vi "xyzt-gui.vi"() -> ()   [LabVIEW 2011]
panel:
  in  "close":bool
  in  "Tab Control":enum32{"Setup", "Run"}(tab)
  in  "start":dbl=0.00262763 min=0.0 max=0.03 step=1e-06 format="%#_6p"
  in  "end":dbl=0.00275375 min=1e-06 max=0.03 step=1e-06 format="%#_6p"
  in  "distance":dbl=1e-05 min=0.0 max=0.0005 step=1e-07 format="%#_6p"
  out "Slices":u16=13
  in  "Get start":bool
  in  "Get end":bool
  in  "Power":T1={"Start-power"=0.02, "double distance"=0.0001} {"double distance" min=0.0 max=0.00025 step=1e-06 format="%#_6p"; "Start-power" format="%#_3p"}
  in  "Frame-time":dbl=1.61596
  in  "z-delay [s]":dbl=0.2 min=0.0 step=0.1
  in  "Get frametime":bool
  in  "xy-positions":dbl[][](array[numeric])=[[0.01555, 0.01516], [0.01923, 0.01332]]
  in  "move time [s]":dbl=2.0
  in  "Add current":bool
  in  "Motors":string[](array[string])=["stage.x", "stage.y"]
  in  "Time":dbl=60.0
  in  "Executions":u32=4
  in  "Calculate fastest":bool
  in  "Experiment-name":string="Z-xy-Time4"
  in  "Run":bool
  in  "cancel":bool
  out "Running":u16[](array[numeric])=[3, 1, 1]
  out "of":u32[](array[numeric])=[13, 2, 4]
  out "wait (time loop)":ext=52.08099985122681
  in  "runstate":enum16{"idle", "run", "cancel", "exit"}(ring)=enum."exit"
  # "First: z-stack"
  # "Second: position or filter"
  # "Third: time-loop"
  # "use u for µm, m for mm"
  # "empty = current only"
  # "Remove:\nRight click on row: Delete Row"
  # "z-loop\n\nmotor-loop\n\ntime-loop"
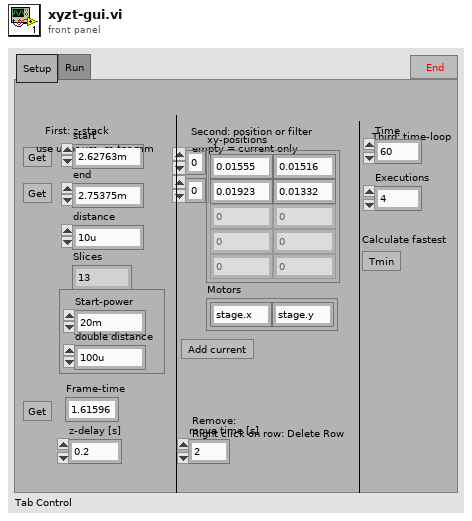
[diagram p1: front panel]
types:
  T1 = cluster{"Start-power":dbl, "double distance":dbl}
  T2 = enum16{"None/#Datasets", "Clear", "TagValueOf#", "AddValues", "ReadValue", "ChangeValue", "Get all"}
  T3 = typedef "ScanControl.ctl" = cluster{"Time [s]":dbl, "action":T4, "channel":T5, "value (/s)":dbl}[]
  T4 = typedef "ScanControl_Action.ctl" = enum16{"Abs", "Rel", "Inc", "IncInc", "LoopStart", "LoopEnd", "WaitTriggerRising"}
  T5 = typedef "ScanControl_Channel.ctl" = enum16{"Com", "AnalogConfig", "AnalogValue", "GalvoX", "GalvoY", "Galvo3", "Galvo4", "Digital", "Free", "Loop", "SMoveTime", "Image1X", "Image1Y", "Image2X", "Image2Y"}
  T6 = cluster{"Time [s]":dbl, "action":T4, "channel":T5, "value (/s)":dbl}
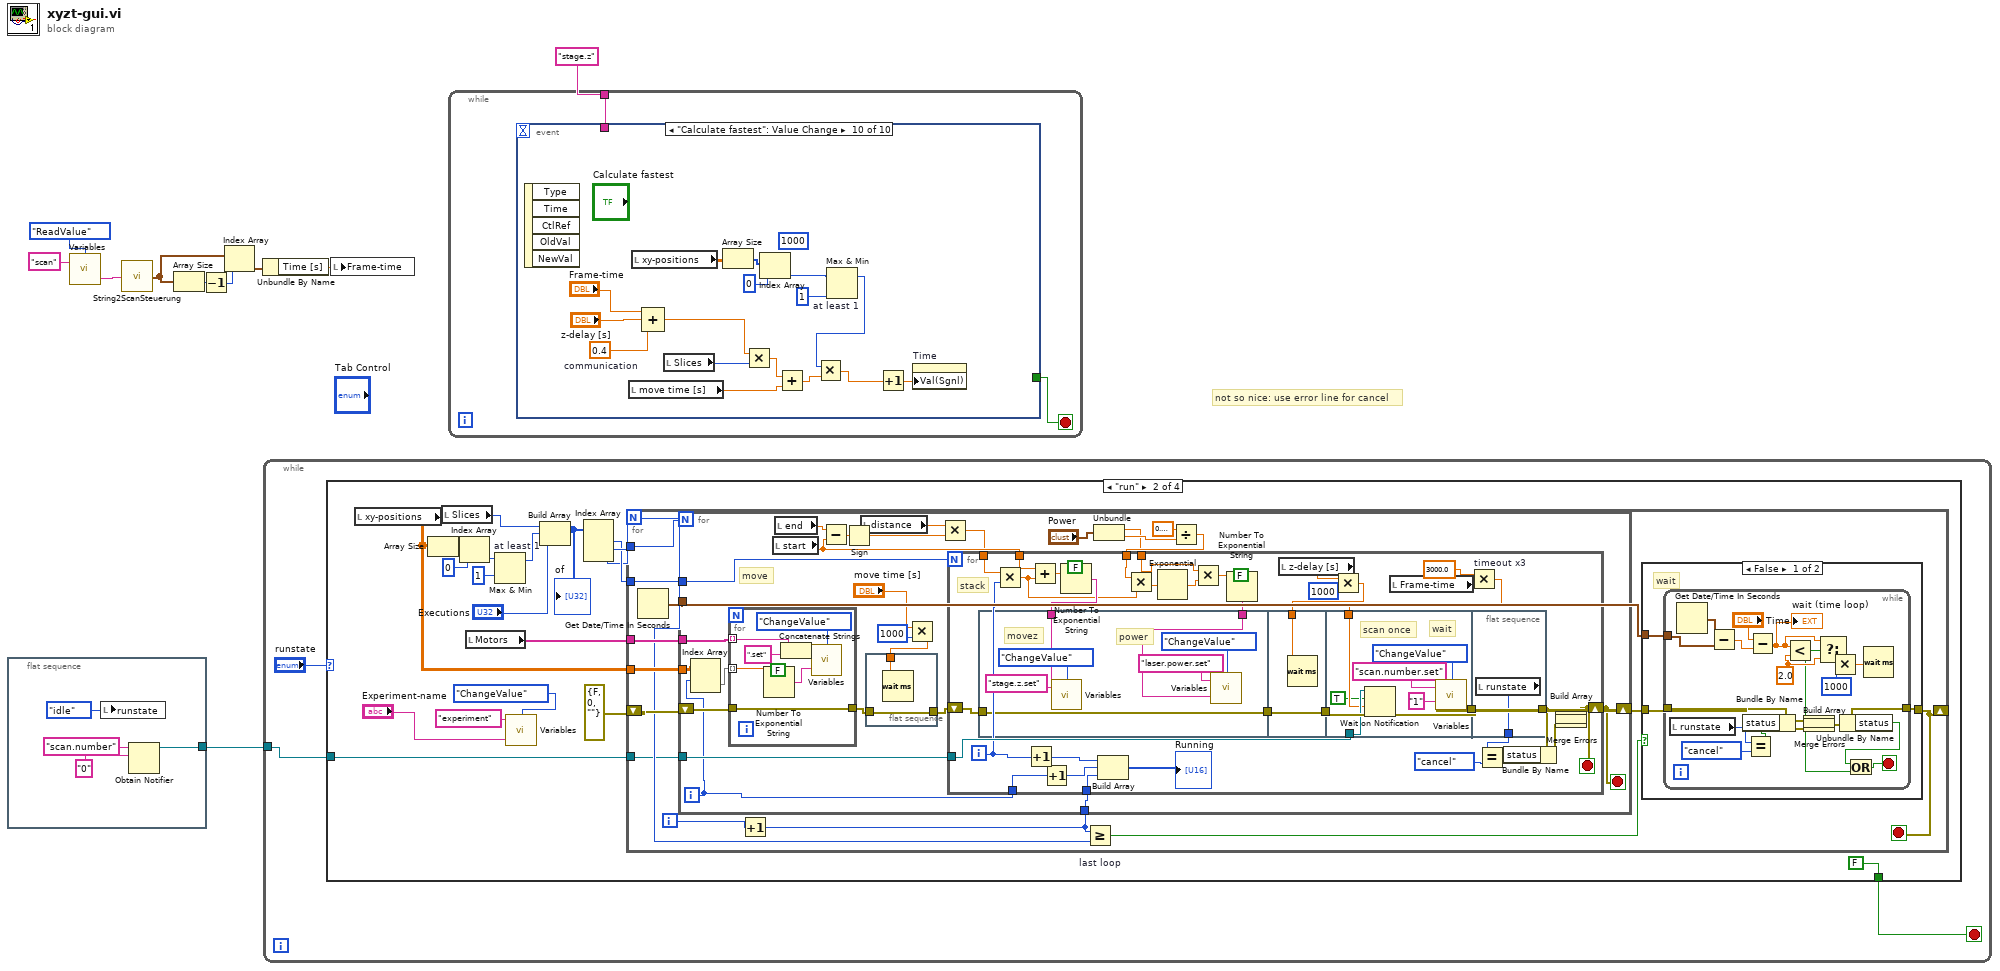
[diagram p0: block diagram]
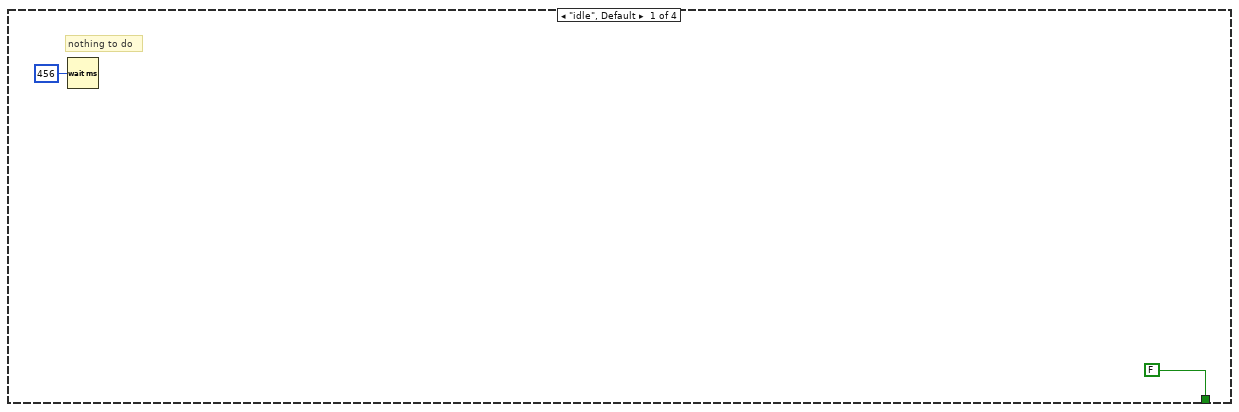
[diagram p2: hidden frame]
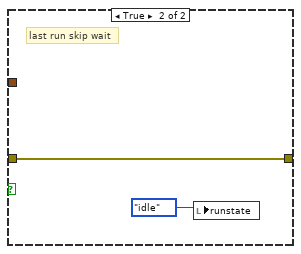
[diagram p3: hidden frame]
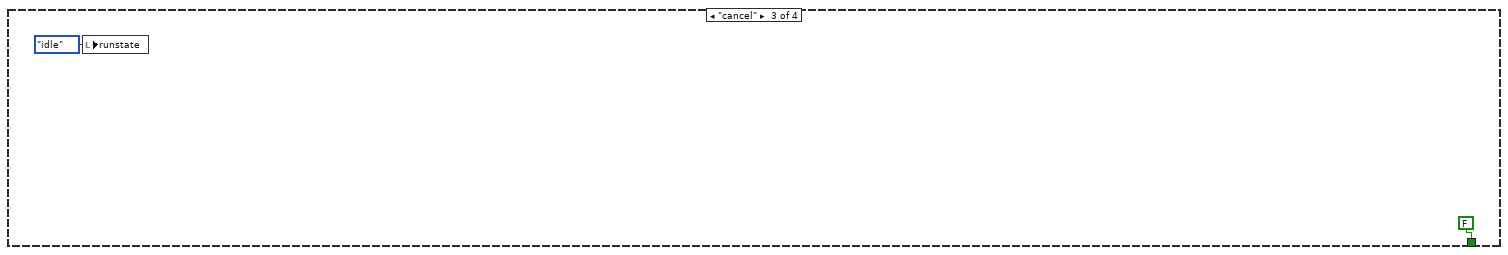
[diagram p4: hidden frame]
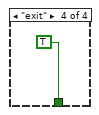
[diagram p5: hidden frame]
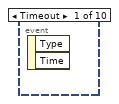
[diagram p6: hidden frame]
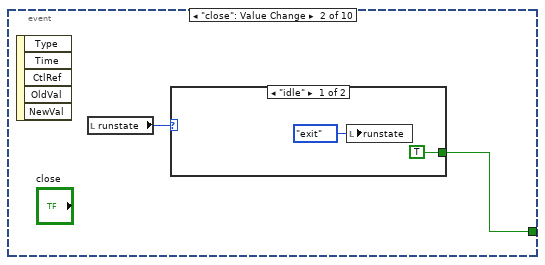
[diagram p7: hidden frame]
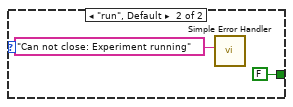
[diagram p8: hidden frame]
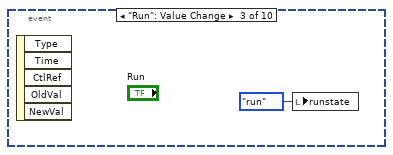
[diagram p9: hidden frame]
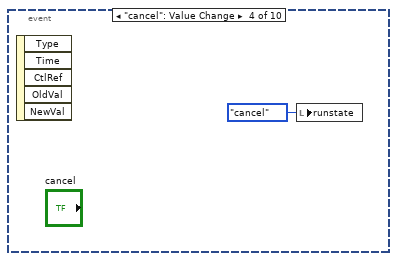
[diagram p10: hidden frame]
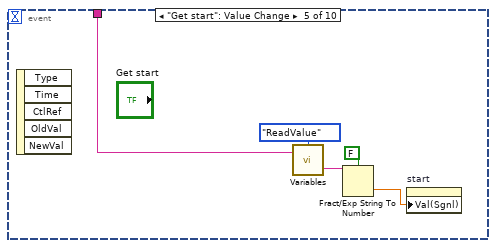
[diagram p11: hidden frame]
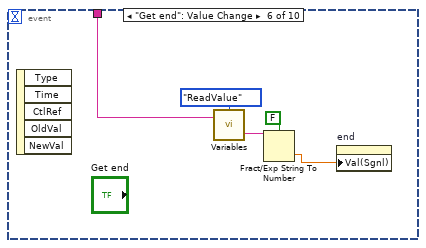
[diagram p12: hidden frame]
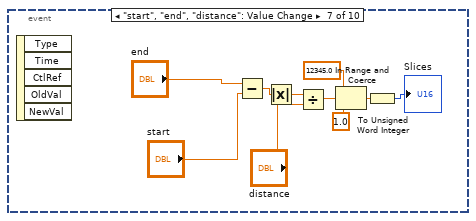
[diagram p13: hidden frame]
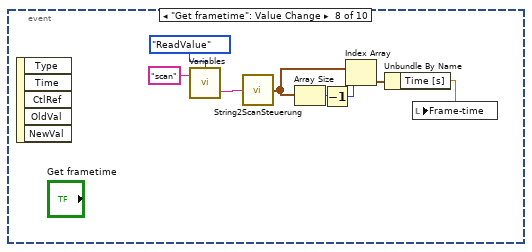
[diagram p14: hidden frame]
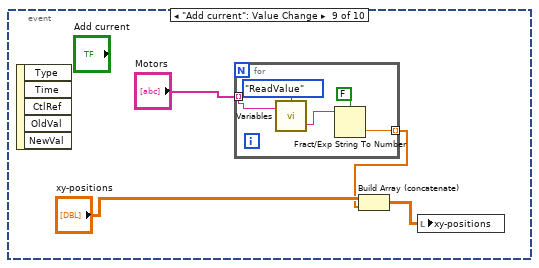
[diagram p15: hidden frame]
diagram:
  # "not so nice: use error line for cancel"
  n1 = flat-sequence {
    tunnel: [w12] -> w9
    frame #0 {
      n2 = local write "runstate"(enum16{"idle", "run", "cancel", "exit"}."idle" ("runstate")) -> ()
      n3 = Obtain Notifier(name (unnamed)="scan.number", notification data type="0") -> (notifier out=w12:refnum<notifier>)  [unwired: 2 in, 2 out]
    }
  }
  n4 = call "Variables.vi"("Tag in"="scan", "Command"=T2."ReadValue") -> ("value out"=w6:string)  [unwired: 1 in, 2 out]
  n5 = call "String2ScanSteuerung.vi"("String"=w6) -> ("ScanSteuerung"=w5:T3)
  n6 = Array Size(array=w5) -> (size(s)=w4:i32)
  n7 = Decrement(x=w4) -> (x-1=w3:i32)
  n8 = Index Array(array=w5, index=w3) -> (element=w2:T6)
  n9 = Unbundle By Name(w2) -> ("Time [s]"=w1:dbl)
  n10 = while {
    tunnel: w9 -> [w17]
    stop <- w15 stop-if-true
    n11 = case shown="\"run\"" "runstate" {
      tunnel: w17 -> [_ w28 _ _]
      tunnel: [FALSE FALSE FALSE TRUE] -> w15
      frame "idle", Default {
        # "nothing to do"
        n12 = Wait (ms)(milliseconds to wait=u32 456) -> ()  [unwired: 1 out]
      }
      frame "run" {
        n13 = local read "xy-positions"() -> (w30:dbl[][])
        n14 = Array Size(array=w30) -> (size(s)=w34:i32[])
        n15 = local read "Slices"() -> (w32:u16)
        n16 = Index Array(array=w34, index=0) -> (element=w22:i32)
        n17 = local read "Motors"() -> (w29:string[])
        n18 = Max & Min "at least 1"(x=w22, y=1) -> (max(x,y)=w20:i32)  [unwired: 1 out]
        n19 = call "Variables.vi"("value"="Experiment-name", "Tag in"="experiment", "Command"=T2."ChangeValue") -> ()  [unwired: 3 out]
        n20 = Build Array(w32, w20, "Executions") -> (w31:u32[])
        "of" <- w31
        n21 = Index Array(array=w31) -> (element #1=w37:u32, element #2=w38:u32, element #3=w36:u32)  [unwired: 3 in]
        n22 = for {
          N: w36 -> [w45]
          tunnel: w38 -> [w51]
          tunnel: w37 -> [w50]
          shift-right: [w43] -> _
          shift-left: errorcluster {"status"=FALSE, "code"=0, "source"=""} ("error constant") -> [w49]
          tunnel: w30 -> [w48]
          tunnel: w29 -> [w47]
          tunnel: w28 -> [w41]
          i -> [w46]
          stop <- w43 stop-if-true
          n23 = Get Date/Time In Seconds() -> (seconds since 1Jan1904=w39:timestamp)
          n24 = Increment(x=w46) -> (x+1=w40:i32)
          n25 = for {
            N: w51 -> [_]
            tunnel: w50 -> [w100]
            shift-right: [w92] -> w44
            shift-left: w49 -> [w95]
            tunnel: w48 -> [w96]
            tunnel: w47 -> [w97]
            tunnel: w39 -> [_]
            tunnel: w41 -> [w91]
            tunnel: w40 -> [w90]
            i -> [w82]
            stop <- w92 stop-if-true
            # "move"
            n26 = Index Array(array=w96, index (row)=w82) -> (element=w83:dbl[])  [unwired: 1 in]
            n27 = for {
              tunnel: w97 -> [w108] mode=indexing
              tunnel: w83 -> [w106] mode=indexing
              tunnel: w95 -> [w110]
              tunnel: [w110] -> w94
              n28 = Number To Exponential String(number=w106, 1:FALSE ("use system decimal point (T)")) -> (E-format string=w105:string)  [unwired: 2 out]
              n29 = Concatenate Strings(w108, ".set" ("string")) -> (w104:string)
              n30 = call "Variables.vi"("value"=w105, "Tag in"=w104, "Command"=T2."ChangeValue") -> ()  [unwired: 3 out]
            }
            n31 = local read "start"() -> (w80:dbl)
            n32 = local read "end"() -> (w81:dbl)
            n33 = Subtract(x=w81, y=w80) -> (x-y=w79:dbl)
            n34 = Sign(1:w79) -> (0:w77:dbl)
            n35 = local read "distance"() -> (w78:dbl)
            n36 = flat-sequence {
              tunnel: w98 -> [w102]
              tunnel: w94 -> [w101]
              tunnel: [w101] -> w93
              frame #0 {
                n37 = Wait (ms)(milliseconds to wait=w102) -> ()  [unwired: 1 out]
              }
            }
            n38 = Multiply(x="move time [s]", y=u32 1000 ("milliseconds to wait")) -> (x*y=w98:dbl)
            n39 = Multiply(x=w78, y=w77) -> (x*y=w76:dbl)
            n40 = Unbundle("Power") -> ("Start-power"=w85:dbl, "double distance"=w87:dbl)
            n41 = Divide(x=0.6931471805599453, y=w87) -> (x/y=w86:dbl)
            n42 = for {
              N: w100 -> [_]
              tunnel: w82 -> [w140]
              tunnel: w90 -> [w147]
              shift-right: [w119] -> w92
              shift-left: w93 -> [w144]
              tunnel: w91 -> [w143]
              tunnel: w76 -> [w139]
              tunnel: w80 -> [w138]
              tunnel: w86 -> [w129]
              tunnel: w85 -> [w128]
              i -> [w114]
              stop <- w119 stop-if-true
              # "stack"
              n43 = flat-sequence {
                tunnel: w144 -> [w154]
                tunnel: [w154] -> w134
                tunnel: w135 -> [w149]
                tunnel: w124 -> [w148]
                tunnel: w134 -> [w156]
                tunnel: [w156] -> w118
                tunnel: w133 -> [w155]
                tunnel: w118 -> [w164]
                tunnel: w143 -> [w162]
                tunnel: w115 -> [w158]
                tunnel: [w163] -> w113
                tunnel: [w166] -> w121
                tunnel: w113 -> [w166]
                tunnel: [w165] -> w112
                frame #0 {
                  # "movez"
                  # "power"
                  n44 = call "Variables.vi"("value"=w149, "Tag in"="stage.z.set", "Command"=T2."ChangeValue") -> ()  [unwired: 3 out]
                  n45 = call "Variables.vi"("value"=w148, "Tag in"="laser.power.set", "Command"=T2."ChangeValue") -> ()  [unwired: 3 out]
                }
                frame #1 {
                  n46 = Wait (ms)(milliseconds to wait=w155) -> ()  [unwired: 1 out]
                }
                frame #2 {
                  # "scan once"
                  # "wait"
                  n47 = Wait on Notification(notifier=w162, ignore previous (F)=TRUE, timeout in ms (-1)=w158, error in (no error)=w164) -> (error out=w163:errorcluster)  [unwired: 3 out]
                  n48 = call "Variables.vi"("value"="1", "Tag in"="scan.number.set", "Command"=T2."ChangeValue") -> ()  [unwired: 3 out]
                }
                frame #3 {
                  n49 = local read "runstate"() -> (w165:enum16{"idle", "run", "cancel", "exit"})
                }
              }
              n50 = Multiply(x=w139, y=w114) -> (x*y=w131:dbl)
              n51 = Increment(x=w114) -> (x+1=w142:i32)
              n52 = Add(x=w138, y=w131) -> (x+y=w137:dbl)
              n53 = Increment(x=w140) -> (x+1=w132:i32)
              n54 = Number To Exponential String(number=w137, 1:FALSE ("use system decimal point (T)")) -> (E-format string=w135:string)  [unwired: 2 out]
              n55 = Build Array(w142, w132, w147) -> (→"Running":i32[])
              n56 = Multiply(x=w129, y=w131) -> (x*y=w130:dbl)
              n57 = Exponential(1:w130) -> (0:w127:dbl)
              n58 = Multiply(x=w128, y=w127) -> (x*y=w125:dbl)
              n59 = Number To Exponential String(number=w125, 1:FALSE ("use system decimal point (T)")) -> (E-format string=w124:string)  [unwired: 2 out]
              n60 = local read "z-delay [s]"() -> (w145:dbl)
              n61 = Multiply(x=w145, y=u32 1000 ("milliseconds to wait")) -> (x*y=w133:dbl)
              n62 = local read "Frame-time"() -> (w117:dbl)
              n63 = Multiply "timeout x3"(x=3000.0, y=w117) -> (x*y=w115:dbl)
              n64 = Equal?(x=w112, y=enum16{"idle", "run", "cancel", "exit"}."cancel" ("runstate")) -> (x = y?=w122:bool)
              n65 = Bundle By Name(cluster=w121, "status"=w122) -> (w120:errorcluster)
              n66 = Build Array(w121, w120) -> (w111:errorcluster[])
              n67 = Merge Errors(w111) -> (w119:errorcluster)
            }
          }
          n68 = Greater Or Equal? "last loop"(x=w40, y=w45) -> (x >= y?=w42:bool)
          n69 = case shown="False" w42 {
            tunnel: w44 -> [w54 w75]
            tunnel: [w53 w75] -> w43
            tunnel: w39 -> [w52 _]
            frame False {
              # "wait"
              n70 = while {
                tunnel: w54 -> [w59]
                tunnel: [w57] -> w53
                tunnel: w52 -> [w71]
                stop <- w64 stop-if-true
                w67 = 2.0 ("upper limit")
                n71 = local read "runstate"() -> (w62:enum16{"idle", "run", "cancel", "exit"})
                n72 = Get Date/Time In Seconds() -> (seconds since 1Jan1904=w70:timestamp)
                n73 = Subtract(x=w70, y=w71) -> (x-y=w69:dbl)
                n74 = Equal?(x=w62, y=enum16{"idle", "run", "cancel", "exit"}."cancel" ("runstate")) -> (x = y?=w61:bool)
                n75 = Bundle By Name(cluster=w59, "status"=w61) -> (w58:errorcluster)
                n76 = Subtract(x="Time", y=w69) -> (x-y=w68:dbl)
                "wait (time loop)" <- w68
                n77 = Less?(x=w68, y=w67) -> (x < y?=w65:bool)
                n78 = Build Array(w59, w58) -> (w55:errorcluster[])
                n79 = Merge Errors(w55) -> (w57:errorcluster)
                n80 = Select(t=w68, s=w65, f=w67) -> (s? t:f=w66:dbl)
                n81 = Multiply(x=w66, y=u32 1000 ("milliseconds to wait")) -> (x*y=w72:dbl)
                n82 = Unbundle By Name(w57) -> ("status"=w56:bool)
                n83 = Or(x=w56, y=w65) -> (x .or. y?=w64:bool)
                n84 = Wait (ms)(milliseconds to wait=w72) -> ()  [unwired: 1 out]
              }
            }
            frame True {
              # "last run skip wait"
              n85 = local write "runstate"(enum16{"idle", "run", "cancel", "exit"}."idle" ("runstate")) -> ()
            }
          }
        }
      }
      frame "cancel" {
        n86 = local write "runstate"(enum16{"idle", "run", "cancel", "exit"}."idle" ("runstate")) -> ()
      }
      frame "exit" {
      }
    }
  }
  n87 = local write "Frame-time"(w1) -> ()
  n88 = while {
    tunnel: "stage.z" ("Tag in") -> [w170]
    stop <- w171 stop-if-true
    n89 = event shown="[9] \"Calculate fastest\": Value Change" {
      selector: _ -> [_ _ _ _ _ _ _ _ _ _]
      dyn-events: _ -> [_ _ _ _ _ _ _ _ _ _]
      timeout: _ -> [_ _ _ _ _ _ _ _ _ _]
      tunnel: [_ w172 _ _ _ _ _ _ _ _] -> w171
      tunnel: w170 -> [_ _ _ _ w181 w186 _ _ _ _]
      event Timeout {
        n90 = event-data() -> ()  [unwired: 3 out]
      }
      event "close": Value Change {
        n91 = event-data() -> ()  [unwired: 6 out]
        n92 = local read "runstate"() -> (w173:enum16{"idle", "run", "cancel", "exit"})
        n93 = case shown="\"idle\"" w173 {
          tunnel: [TRUE FALSE] -> w172
          frame "idle" {
            n94 = local write "runstate"(enum16{"idle", "run", "cancel", "exit"}."exit" ("runstate")) -> ()
          }
          frame "run", Default {
            n95 = call <vilib>:"Simple Error Handler.vi"("error source (\" \")"="Can not close: Experiment running" ("error source (\" \")")) -> ()  [unwired: 2 in, 7 out]
          }
        }
      }
      event "Run": Value Change {
        n96 = event-data() -> ()  [unwired: 6 out]
        n97 = local write "runstate"(enum16{"idle", "run", "cancel", "exit"}."run" ("runstate")) -> ()
      }
      event "cancel": Value Change {
        n98 = event-data() -> ()  [unwired: 6 out]
        n99 = local write "runstate"(enum16{"idle", "run", "cancel", "exit"}."cancel" ("runstate")) -> ()
      }
      event "Get start": Value Change {
        n100 = event-data() -> ()  [unwired: 6 out]
        n101 = call "Variables.vi"("Tag in"=w181, "Command"=T2."ReadValue") -> ("value out"=w183:string)  [unwired: 1 in, 2 out]
        n102 = Fract/Exp String To Number(use system decimal point (T)=FALSE, string=w183) -> (number=w180:dbl)  [unwired: 3 out]
        n103 = property on="start" class="DigNum (strict)"("Val(Sgnl)"=w180) -> ()  [unwired: 2 in, 2 out]
      }
      event "Get end": Value Change {
        n104 = event-data() -> ()  [unwired: 6 out]
        n105 = call "Variables.vi"("Tag in"=w186, "Command"=T2."ReadValue") -> ("value out"=w188:string)  [unwired: 1 in, 2 out]
        n106 = Fract/Exp String To Number(use system decimal point (T)=FALSE, string=w188) -> (number=w185:dbl)  [unwired: 3 out]
        n107 = property on="end" class="DigNum (strict)"("Val(Sgnl)"=w185) -> ()  [unwired: 2 in, 2 out]
      }
      event "start", "end", "distance": Value Change {
        n108 = event-data() -> ()  [unwired: 6 out]
        n109 = Subtract(x="end", y="start") -> (x-y=w191:dbl)
        n110 = Absolute Value(x=w191) -> (abs(x)=w190:dbl)
        n111 = Divide(x=w190, y="distance") -> (x/y=w195:dbl)
        n112 = In Range and Coerce(upper limit=12345.0, x=w195, lower limit=1.0) -> (coerced(x)=w194:dbl)  [unwired: 1 out]
        n113 = To Unsigned Word Integer(number=w194) -> (unsigned 16bit integer=→"Slices":u16)
      }
      event "Get frametime": Value Change {
        n114 = event-data() -> ()  [unwired: 6 out]
        n115 = call "Variables.vi"("Tag in"="scan", "Command"=T2."ReadValue") -> ("value out"=w205:string)  [unwired: 1 in, 2 out]
        n116 = call "String2ScanSteuerung.vi"("String"=w205) -> ("ScanSteuerung"=w204:T3)
        n117 = Array Size(array=w204) -> (size(s)=w203:i32)
        n118 = Decrement(x=w203) -> (x-1=w202:i32)
        n119 = Index Array(array=w204, index=w202) -> (element=w201:T6)
        n120 = Unbundle By Name(w201) -> ("Time [s]"=w200:dbl)
        n121 = local write "Frame-time"(w200) -> ()
      }
      event "Add current": Value Change {
        n122 = event-data() -> ()  [unwired: 6 out]
        n123 = for {
          tunnel: "Motors" -> [w215] mode=indexing
          tunnel: [w212] -> w209 mode=indexing
          n124 = call "Variables.vi"("Tag in"=w215, "Command"=T2."ReadValue") -> ("value out"=w213:string)  [unwired: 1 in, 2 out]
          n125 = Fract/Exp String To Number(use system decimal point (T)=FALSE, string=w213) -> (number=w212:dbl)  [unwired: 3 out]
        }
        n126 = Build Array (concatenate)("xy-positions", w209) -> (w208:dbl[][])
        n127 = local write "xy-positions"(w208) -> ()
      }
      event "Calculate fastest": Value Change {
        w220 = 0.4  # communication
        (unwired) 1000 ("upper limit")
        n128 = event-data() -> ()  [unwired: 6 out]
        n129 = local read "move time [s]"() -> (w226:dbl)
        n130 = local read "xy-positions"() -> (w229:dbl[][])
        n131 = Compound Arithmetic op=ADD("Frame-time", "z-delay [s]", w220) -> (w230:dbl)
        n132 = local read "Slices"() -> (w232:u16)
        n133 = Array Size(array=w229) -> (size(s)=w228:i32[])
        n134 = Multiply(x=w230, y=w232) -> (x*y=w225:dbl)
        n135 = Index Array(array=w228, index=0) -> (element=w218:i32)
        n136 = Add(x=w225, y=w226) -> (x+y=w224:dbl)
        n137 = Max & Min "at least 1"(x=w218, y=1 ("lower limit")) -> (max(x,y)=w217:i32)  [unwired: 1 out]
        n138 = Multiply(x=w217, y=w224) -> (x*y=w223:dbl)
        n139 = Increment(x=w223) -> (x+1=w222:dbl)
        n140 = property on="Time" class="DigNum (strict)"("Val(Sgnl)"=w222) -> ()  [unwired: 2 in, 2 out]
      }
    }
  }
